vi "hse-application_DetermineProgramInfo.vi"(5 "Project Name":string, 7 "Project Folder":path, 8 "error in":errorcluster, 11 "Application in":refnum<class "hse-application.lvclass">) -> (0 "error out":errorcluster, 3 "Application out":refnum<class "hse-application.lvclass">)   [LabVIEW 2014, in "hse-application.lvclass"]
doc: "____\nHAMPEL SOFTWARE ENGINEERING v0.12.0 (2018-09-13 18:21)"
uses:
  hse-application.lvclass
  hse-application.lvclass/hse-application.ctl
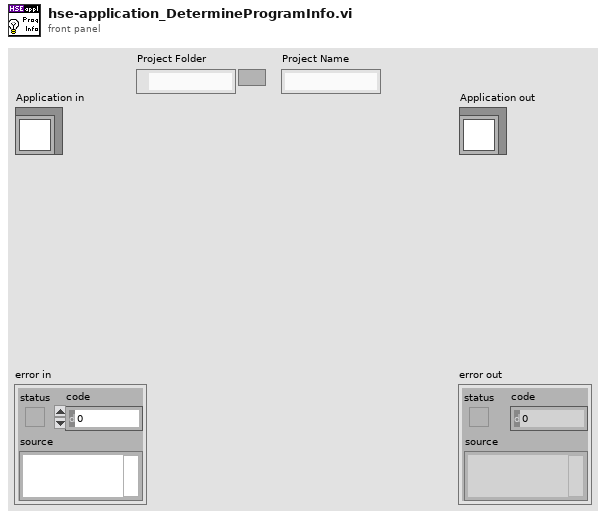
[diagram p1: front panel]
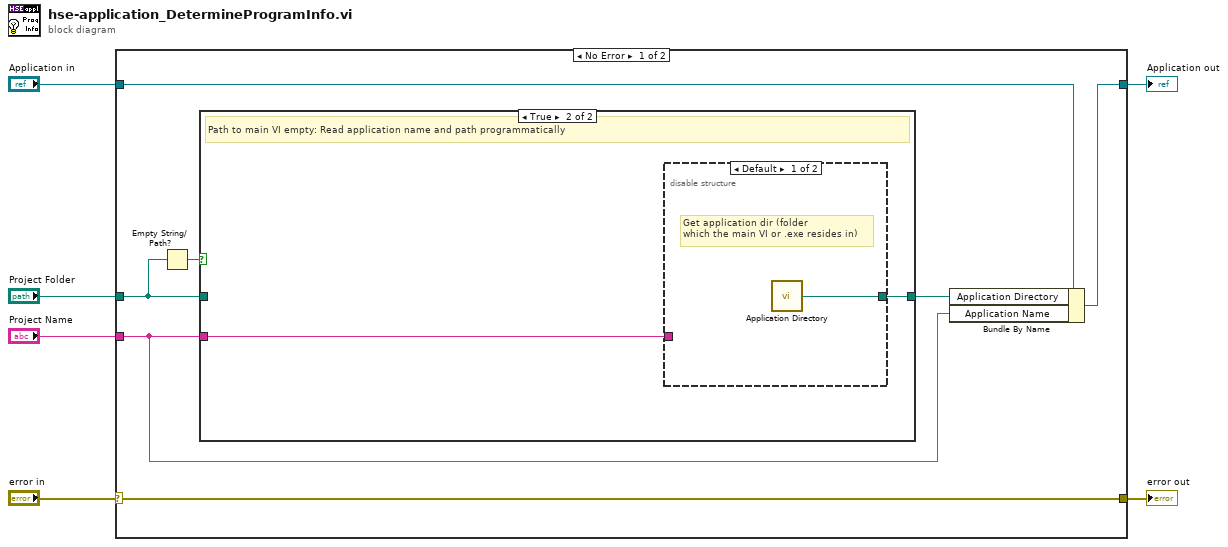
[diagram p0: block diagram]
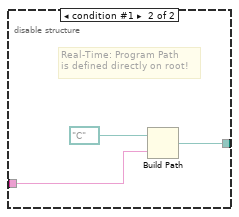
[diagram p3: hidden frame]
diagram:
  n1 = case shown="No Error" "error in" {
    selector: "error in" -> [w10 w21]
    tunnel: [w10 w21] -> w5
    tunnel: [w12 w22] -> w3
    tunnel: "Application in" -> [w13 w22]
    tunnel: "Project Folder" -> [w8 _]
    tunnel: "Project Name" -> [w7 _]
    frame No Error {
      n2 = Empty String/Path?(string/path=w8) -> (empty?=w9:bool)
      n3 = case shown="True" w9 {
        tunnel: [w14 w16] -> w11
        tunnel: w8 -> [w14 _]
        tunnel: w7 -> [_ w15]
        frame False {
          # "Path to main VI not empty: Take application name and path from that value"
        }
        frame True {
          # "Path to main VI empty: Read application name and path programmatically"
          n4 = disable-structure shown="Default" {
            disable-tunnel: [w17 w20] -> w16
            disable-tunnel: w15 -> [_ w18]
            frame condition #0 (active) {
              # "Get application dir (folder \nwhich the main VI or .exe resides in)"
              n5 = call <vilib>:"Application Directory.vi"() -> ("Application Directory"=w17:path)
            }
            frame condition #1 {
              # "Real-Time: Program Path\nis defined directly on root!"
              n6 = Build Path(base path=path "C:/" ("Path Program"), name or relative path=w18) -> (appended path=w20:path)
            }
          }
        }
      }
      n7 = Bundle By Name(cluster=w13, "Application Directory"=w11, "Application Name"=w7) -> (w12:refnum<class "hse-application.lvclass">)
    }
    frame Error {
    }
  }
  "error out" <- w5
  "Application out" <- w3
